vi "Protoc UI Create Project.vi"(11 "Output Folder":path) -> ()   [LabVIEW 2020]
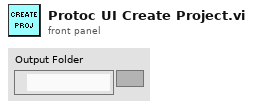
[diagram p1: front panel]
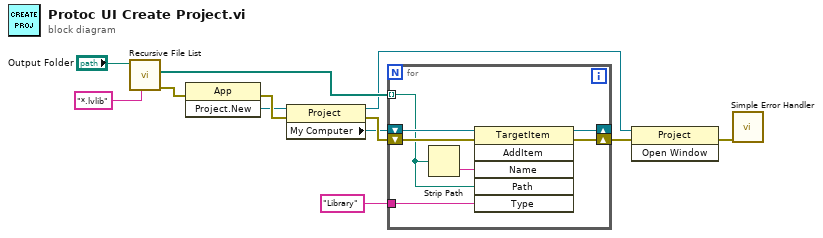
[diagram p0: block diagram]
diagram:
  n1 = call <vilib>:"Recursive File List.vi"("pattern"="*.lvlib", "Folder Path"="Output Folder") -> ("error out"=w5:errorcluster, "All Files in Dir"=w8:path[])  [unwired: 5 in, 3 out]
  n2 = invoke class="App" method="Project.New"(error in=w5) -> (error out=w11:errorcluster, "Project:New"=w7:refnum<vi>)  [unwired: 2 in, 1 out]
  n3 = property class="Project"(reference=w7, error in=w11) -> (reference out=w3:refnum<vi>, error out=w12:errorcluster, "My Computer"=w6:refnum<vi>)
  n4 = for {
    tunnel: w8 -> [w14] mode=indexing
    shift-right: [w18] -> _
    shift-left: w6 -> [w19]
    shift-right: [w16] -> w4
    shift-left: w12 -> [w17]
    tunnel: "Library" -> [w15]
    n5 = Strip Path(path=w14) -> (name=w13:string)  [unwired: 1 out]
    n6 = invoke class="TargetItem" method="AddItem"(reference=w19, error in=w17, "Name"=w13, "Path"=w14, "Type"=w15) -> (reference out=w18:refnum<vi>, error out=w16:errorcluster)  [unwired: 1 in, 4 out]
  }
  n7 = invoke class="Project" method="Open Window"(reference=w3, error in=w4) -> (error out=w2:errorcluster)  [unwired: 1 in, 2 out]
  n8 = call <vilib>:"Simple Error Handler.vi"("error in (no error)"=w2) -> ()  [unwired: 4 in, 5 out]
